vi "solar_voy_def Resolve IDs.vi"(7 "VoyagerIDOffset":u16, 10 "PACKETS in":T1[](array[typedef]) {"last_time" format="%<%H:%M:%S%3u %m/%d/%y>T"}) -> (2 "PACKETS out":T1[](array[typedef]) {"last_time" format="%<%H:%M:%S%3u %m/%d/%y>T"})   [LabVIEW 2018]
doc: "This creates a new packet ID if the ID is 0. To account for custom ICD files, Voyager packet IDs start at 10000. All IDs must be unique for a given LINC interface."
uses:
  solar_voy_def_ctl ITEM TYPE.ctl
  type/solar_type Item Type.ctl
  solar_voy_def_ctl ITEM.ctl
  solar_voy_def_ctl PACKET_ID.ctl
  solar_voy_def_ctl PACKET.ctl
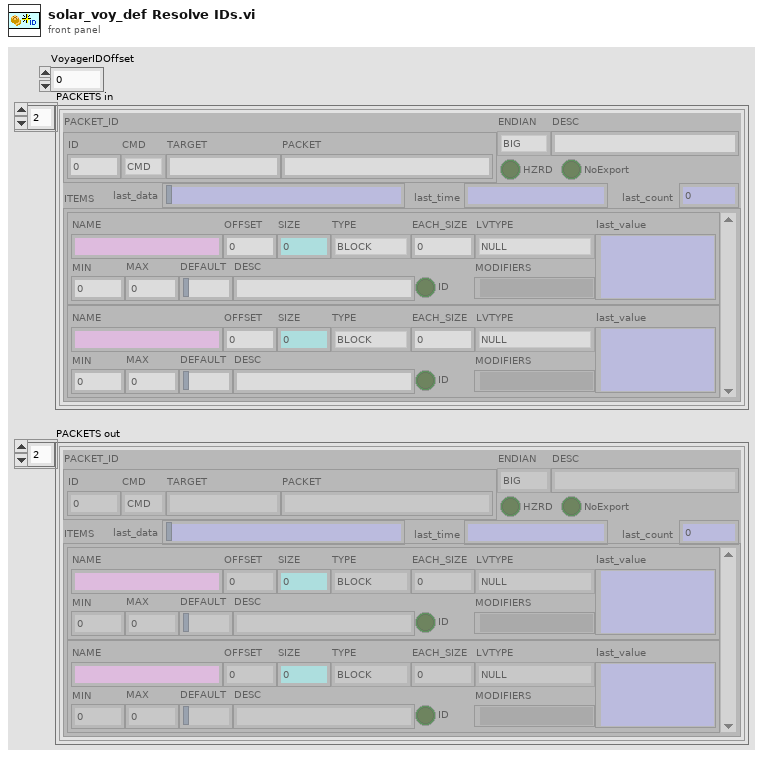
[diagram p1: front panel]
types:
  T1 = typedef "solar_voy_def_ctl PACKET.ctl" = cluster{"PACKET_ID":T2, "ENDIAN":enum8{"BIG", "LITTLE"}, "DESC":string, "HZRD":bool, "ITEMS":T3[], "NoExport":bool, "last_time":timestamp, "last_count":u32, "last_data":string}
  T2 = typedef "solar_voy_def_ctl PACKET_ID.ctl" = cluster{"ID":u16, "CMD":enum8{"CMD", "TLM"}, "TARGET":string, "PACKET":string}
  T3 = typedef "solar_voy_def_ctl ITEM.ctl" = cluster{"NAME":string, "OFFSET":i32, "SIZE":i32, "TYPE":T4, "EACH_SIZE":i32, "LVTYPE":T5, "MIN":dbl, "MAX":dbl, "DEFAULT":string, "DESC":string, "ID":bool, "MODIFIERS":variant, "last_value":variant}
  T4 = typedef "solar_voy_def_ctl ITEM TYPE.ctl" = enum8{"BLOCK", "INT", "UINT", "FLOAT", "STRING"}
  T5 = typedef "solar_type Item Type.ctl" = enum16{"NULL", "UNKNOWN", "CLUSTER", "I8", "I16", "I32", "I64", "U8", "U16", "U32", "U64", "U8_ENUM", "U16_ENUM", "U32_ENUM", "SGL", "DBL", "BOOLEAN", "STRING", "PATH", "VISA", "TAG", "TIME", "I8_1D", "I16_1D", "I32_1D", "I64_1D", "U8_1D", "U16_1D", "U32_1D", "U64_1D", "U8_ENUM_1D", "U16_ENUM_1D", "U32_ENUM_1D", "SGL_1D", "DBL_1D", "BOOLEAN_1D", "STRING_1D", "PATH_1D", "VISA_1D", "TAG_1D", "TIME_1D", "I8_2D", "I16_2D", "I32_2D", "I64_2D", "U8_2D", "U16_2D", "U32_2D", "U64_2D", "U8_ENUM_2D", "U16_ENUM_2D", "U32_ENUM_2D", "SGL_2D", "DBL_2D", "BOOLEAN_2D", "STRING_2D", "PATH_2D", "VISA_2D", "TAG_2D", "TIME_2D"}
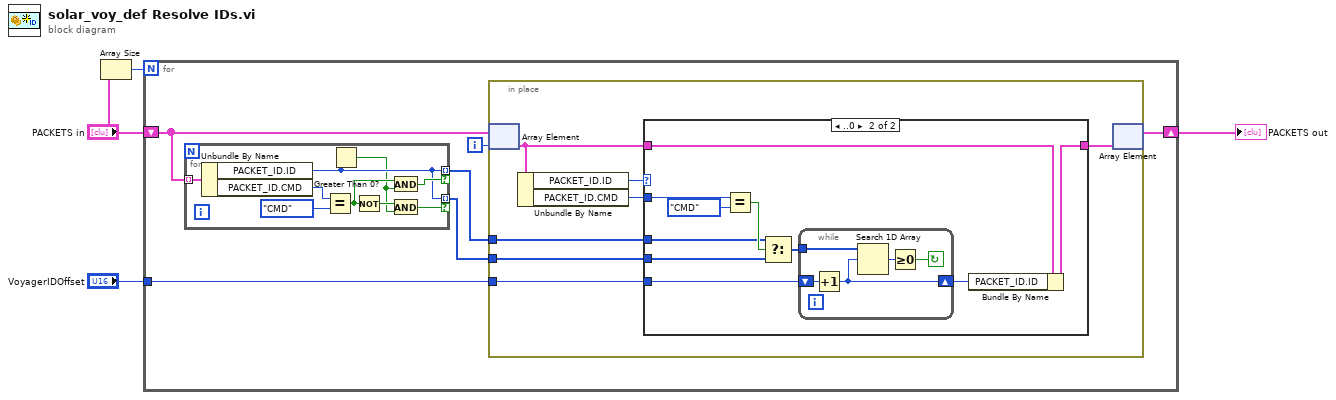
[diagram p0: block diagram]
diagram:
  n1 = Array Size(array="PACKETS in") -> (size(s)=w2:i32)
  n2 = for {
    N: w2 -> [_]
    tunnel: "VoyagerIDOffset" -> [w10]
    shift-right: [w9] -> w4
    shift-left: "PACKETS in" -> [w8]
    i -> [w7]
    n3 = for {
      tunnel: w8 -> [w16] mode=indexing
      tunnel: [w12] -> w6 mode=indexing if=w13
      tunnel: [w12] -> w5 mode=indexing if=w14
      n4 = Unbundle By Name(w16) -> ("PACKET_ID.ID"=w12:u16, "PACKET_ID.CMD"=w19:enum8{"CMD", "TLM"})
      n5 = Equal?(x=w19, y=enum8{"CMD", "TLM"}."CMD") -> (x = y?=w17:bool)
      n6 = Greater Than 0?(x=w12) -> (x > 0?=w11:bool)
      n7 = Not(x=w17) -> (.not. x?=w15:bool)
      n8 = And(x=w17, y=w11) -> (x .and. y?=w13:bool)
      n9 = And(x=w15, y=w11) -> (x .and. y?=w14:bool)
    }
    n10 = in-place {
      in-place-border: w6 -> [w25]
      in-place-border: w5 -> [w24]
      in-place-border: w10 -> [w22]
      n11 = in-place-array #1(w8, w7) -> (w21:T1)
      n12 = Unbundle By Name(w21) -> ("PACKET_ID.ID"=w23:u16, "PACKET_ID.CMD"=w26:enum8{"CMD", "TLM"})
      n13 = case shown="..0" w23 {
        tunnel: w26 -> [_ w36]
        tunnel: w25 -> [_ w34]
        tunnel: w24 -> [_ w33]
        tunnel: [w27 w31] -> w20
        tunnel: w21 -> [w27 w32]
        tunnel: w22 -> [_ w29]
        frame 1.. {
        }
        frame ..0 {
          n14 = Equal?(x=w36, y=enum8{"CMD", "TLM"}."CMD") -> (x = y?=w35:bool)
          n15 = Select(t=w34, s=w35, f=w33) -> (s? t:f=w30:u16[])
          n16 = while {
            tunnel: w30 -> [w42]
            shift-right: [w40] -> w28
            shift-left: w29 -> [w41]
            stop <- w38 continue-if-true
            n17 = Increment(x=w41) -> (x+1=w40:u16)
            n18 = Search 1D Array(1D array=w42, element=w40) -> (index of element=w39:i32)  [unwired: 1 in]
            n19 = Greater Or Equal To 0?(x=w39) -> (x >= 0?=w38:bool)
          }
          n20 = Bundle By Name(cluster=w32, "PACKET_ID.ID"=w28) -> (w31:T1)
        }
      }
      n21 = in-place-array #1(w20) -> (w9:T1[])  [unwired: 1 out]
    }
  }
  "PACKETS out" <- w4
